vi "Simulation iRobot Sensors.vi"(8 "error in":errorcluster, 11 "simulator":T11={"configuration"={"maxTime"=5.0, "enableVisualization"=TRUE, "statechart"=path "iRobot Navigation State Machine.vi", "environment"=path "simulation configuration.ini", "record"=path "Simulation Record.xml", "autograde?"=TRUE, "interactive?"=FALSE, "feedback mode"=enum."debug navigation"}, "Bump Sensors"=[], "Distance Sensors"=[], "Accelerometer"=refnum, "Wall Sensor"=refnum, "Statechart\ndisplay"=refnum, "Body"=refnum, "Left Motor"=refnum, "Right Motor"=refnum, "first step?"=FALSE}) -> (0 "error out":errorcluster, 2 "sensors":T1={"net distance (mm)"=0, "net angle (deg)"=0, "accelerometer"={"x axis (g)"=0.0, "y axis (g)"=0.0, "z axis (g)"=0.0}, "iRobot Sensors"={"Bumps + Wheel Drops"={"Wheeldrop Caster"=FALSE, "Wheeldrop Left"=FALSE, "Wheeldrop Right"=FALSE, "Bump Left"=FALSE, "Bump Right"=FALSE}, "Wall"=FALSE, "Cliff Left"=FALSE, "Cliff Front Left"=FALSE, "Cliff Front Right"=FALSE, "Cliff Right"=FALSE, "Wall Signal"=0, "Cliff Left Signal"=0, "Cliff Front Left Signal"=0, "Cliff Front Right Signal"=0, "Cliff Right Signal"=0, "Buttons"={"Advance"=FALSE, "Play"=FALSE}, "Virtual Wall"=FALSE, "# Stream Packets"=0, "Requested Velocity (mm/s)"=0, "Requested Radius (mm)"=0, "Requested Right Wheel Velocity (mm/s)"=0, "Requested Left Wheel Velocity (mm/s)"=0, "Distance (mm)"=0, "Angle (deg)"=0, "Song Playing"=FALSE, "Song Number"=0, "Charging State"=enum."Not Charging", "Voltage (mV)"=0, "Current (mA)"=0, "Battery Temperature (deg C)"=0, "Battery Charge (mAh)"=0, "Battery Capacity (mAh)"=0, "Charging Sources"={"Internal Charger"=FALSE, "Home Base"=FALSE}, "OI Mode"=enum."Off", "Digital Inputs"={"Digital Input 0"=FALSE, "Digital Input 1"=FALSE, "Digital Input 2"=FALSE, "Digital Input 3"=FALSE, "Device Detect"=FALSE}, "Drivers & Wheel Overcurrent"={"Low-Side Driver 0"=FALSE, "Low-Side Driver 1"=FALSE, "Low-Side Driver 2"=FALSE, "Left Wheel"=FALSE, "Right Wheel"=FALSE}, "Analog Signal"=0, "Infrared"=255}, "Is Simulator?"=FALSE} {"iRobot Sensors"."Infrared" format="%02x"; "accelerometer"."z axis (g)" format="%.3f"; "accelerometer"."y axis (g)" format="%.3f"; "accelerometer"."x axis (g)" format="%.3f"}, 3 "simulator":T11={"configuration"={"maxTime"=5.0, "enableVisualization"=TRUE, "statechart"=path "iRobot Navigation State Machine.vi", "environment"=path "simulation configuration.ini", "record"=path "Simulation Record.xml", "autograde?"=TRUE, "interactive?"=FALSE, "feedback mode"=enum."debug navigation"}, "Bump Sensors"=[], "Distance Sensors"=[], "Accelerometer"=refnum, "Wall Sensor"=refnum, "Statechart\ndisplay"=refnum, "Body"=refnum, "Left Motor"=refnum, "Right Motor"=refnum, "first step?"=FALSE})   [LabVIEW 2013]
doc: "Simulates iRobot sensors. Automatically accumulates distance and angle."
uses:
  Simulator.ctl
  <instrlib>/DC Motor Controller/HAIOL/DC Motor Controller.lvclass
  CyberSim interface/Simulation Configuration.ctl
  autograder/feedbackMode.ctl
  shared/Sensors.ctl
  iRobot/Sensor/Accelerometer.ctl
  iRobot/Sensor/Sensor Group 6.ctl
  iRobot/Sensor/Bumps + Wheel Drops.ctl
  iRobot/Sensor/Buttons.ctl
  iRobot/Sensor/Charging State.ctl
  iRobot/Sensor/Charging Sources Available.ctl
  iRobot/Sensor/OI Mode.ctl
  iRobot/Sensor/Cargo Bay Digital Inputs.ctl
  iRobot/Sensor/Low-Side Driver + Wheel Overcurrent.ctl
  <vilib>/Analysis/coordinate.llb/Angle Units.ctl
  <vilib>/Analysis/coordinate.llb/Wrap Angle (scalar).vi
  <vilib>/Analysis/coordinate.llb/2D Cartesian Coordinate Rotation (Scalar).vi
  <vilib>/Analysis/BLAS.llb/dnrm2 - Vector 2-Norm (DBL).vi
  <resource>/objmgr/LVODE.rc
  <vilib>/Analysis/NI_AALBLAS.lvlib
  <vilib>/robotics/Kinematics/NI_Kinematics.lvlib
  <vilib>/Analysis/NI_AAL_Angle.lvlib
  <vilib>/Analysis/NI_AALPro.lvlib
panel:
  # "Electrical: charging, battery, OI mode"
  # "Sensors: bump, cliff, button, wheel drop, wall, virtual wall"
  # "Motion: distance, angle, requested velocity"
  # "Cargo Bay: I/O, overcurrent, infrared"
  # "Song"
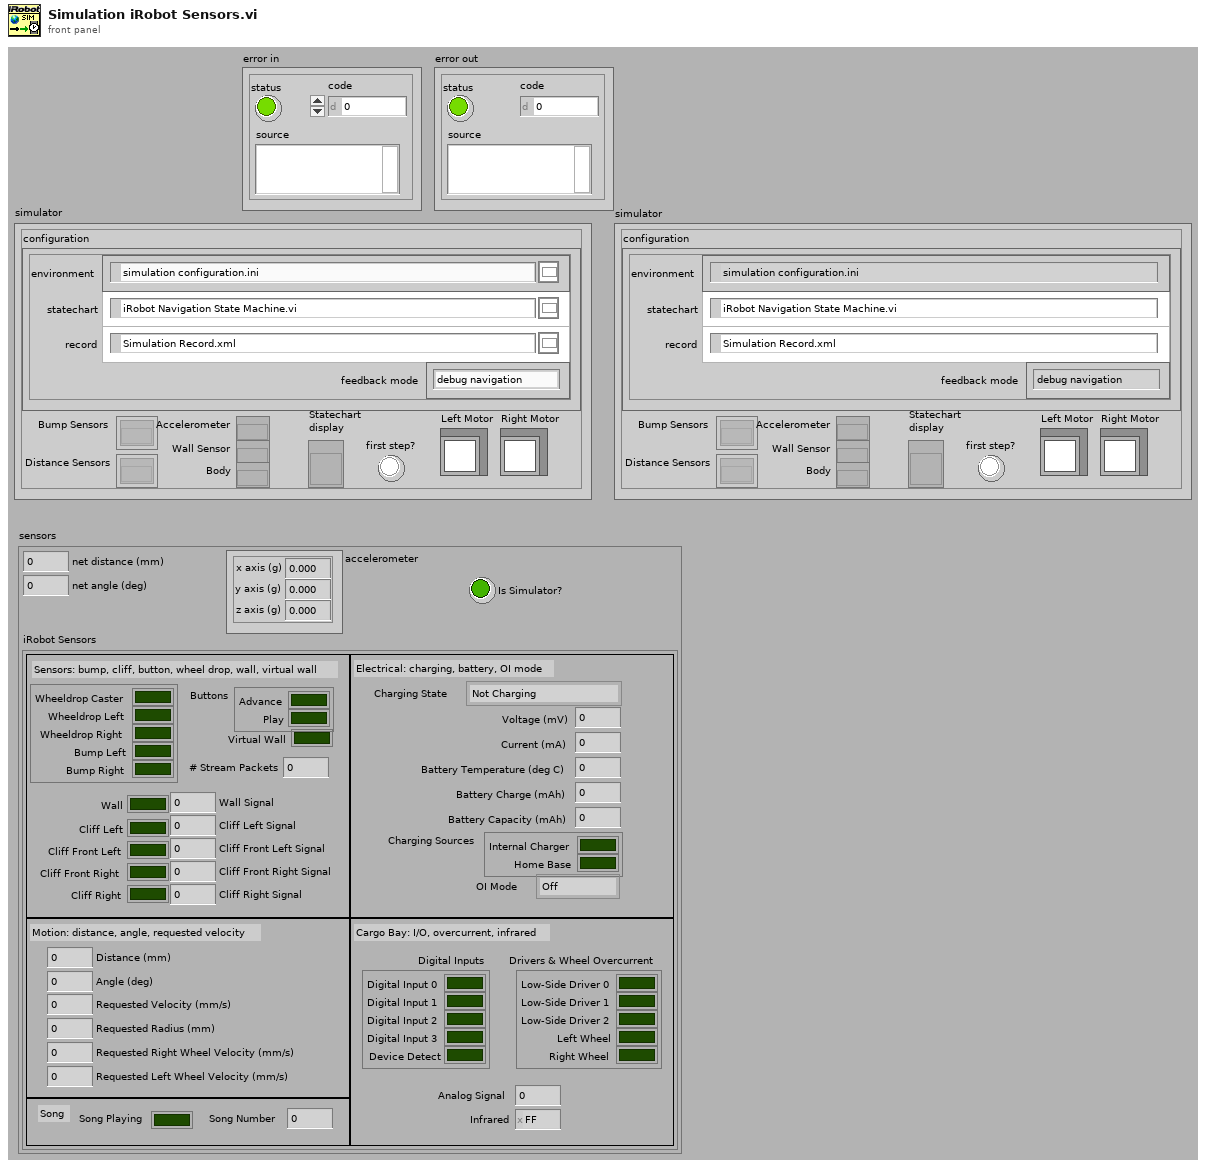
[diagram p1: front panel]
types:
  T1 = typedef "Sensors.ctl" = cluster{"net distance (mm)":i32, "net angle (deg)":i32, "accelerometer":T2, "iRobot Sensors":T3, "Is Simulator?":bool}
  T2 = typedef "Accelerometer.ctl" = cluster{"x axis (g)":dbl, "y axis (g)":dbl, "z axis (g)":dbl}
  T3 = typedef "Sensor Group 6.ctl" = cluster{"Bumps + Wheel Drops":T4, "Wall":bool, "Cliff Left":bool, "Cliff Front Left":bool, "Cliff Front Right":bool, "Cliff Right":bool, "Wall Signal":u16, "Cliff Left Signal":u16, "Cliff Front Left Signal":u16, "Cliff Front Right Signal":u16, "Cliff Right Signal":u16, "Buttons":T5, "Virtual Wall":bool, "# Stream Packets":u8, "Requested Velocity (mm/s)":i16, "Requested Radius (mm)":i16, "Requested Right Wheel Velocity (mm/s)":i16, "Requested Left Wheel Velocity (mm/s)":i16, "Distance (mm)":i32, "Angle (deg)":i32, "Song Playing":bool, "Song Number":u8, "Charging State":T6, "Voltage (mV)":u16, "Current (mA)":i16, "Battery Temperature (deg C)":i8, "Battery Charge (mAh)":u16, "Battery Capacity (mAh)":u16, "Charging Sources":T7, "OI Mode":T8, "Digital Inputs":T9, "Drivers & Wheel Overcurrent":T10, "Analog Signal":u16, "Infrared":u8}
  T4 = typedef "Bumps + Wheel Drops.ctl" = cluster{"Wheeldrop Caster":bool, "Wheeldrop Left":bool, "Wheeldrop Right":bool, "Bump Left":bool, "Bump Right":bool}
  T5 = typedef "Buttons.ctl" = cluster{"Advance":bool, "Play":bool}
  T6 = typedef "Charging State.ctl" = enum16{"Not Charging", "Reconditioning Charging", "Full Charging", "Trickle Charging", "Waiting", "Charging Fault Condition"}
  T7 = typedef "Charging Sources Available.ctl" = cluster{"Internal Charger":bool, "Home Base":bool}
  T8 = typedef "OI Mode.ctl" = enum16{"Off", "Passive", "Safe", "Full"}
  T9 = typedef "Cargo Bay Digital Inputs.ctl" = cluster{"Digital Input 0":bool, "Digital Input 1":bool, "Digital Input 2":bool, "Digital Input 3":bool, "Device Detect":bool}
  T10 = typedef "Low-Side Driver + Wheel Overcurrent.ctl" = cluster{"Low-Side Driver 0":bool, "Low-Side Driver 1":bool, "Low-Side Driver 2":bool, "Left Wheel":bool, "Right Wheel":bool}
  T11 = typedef "Simulator.ctl" = cluster{"configuration":T12, "Bump Sensors":refnum<k20>[], "Distance Sensors":refnum<k20>[], "Accelerometer":refnum<k20>, "Wall Sensor":refnum<k20>, "Statechart\ndisplay":refnum<vi>, "Body":refnum<k20>, "Left Motor":refnum<class "DC Motor Controller.lvclass">, "Right Motor":refnum<class "DC Motor Controller.lvclass">, "first step?":bool}
  T12 = typedef "Simulation Configuration.ctl" = cluster{"maxTime":sgl, "enableVisualization":bool, "statechart":path, "environment":path, "record":path, "autograde?":bool, "interactive?":bool, "feedback mode":T13}
  T13 = typedef "feedbackMode.ctl" = enum32{"debug navigation", "debug hill climb", "autograde navigation", "autograde hill climb"}
  T14 = typedef "NI_AAL_Angle.lvlib/Angle Units.ctl" = i32
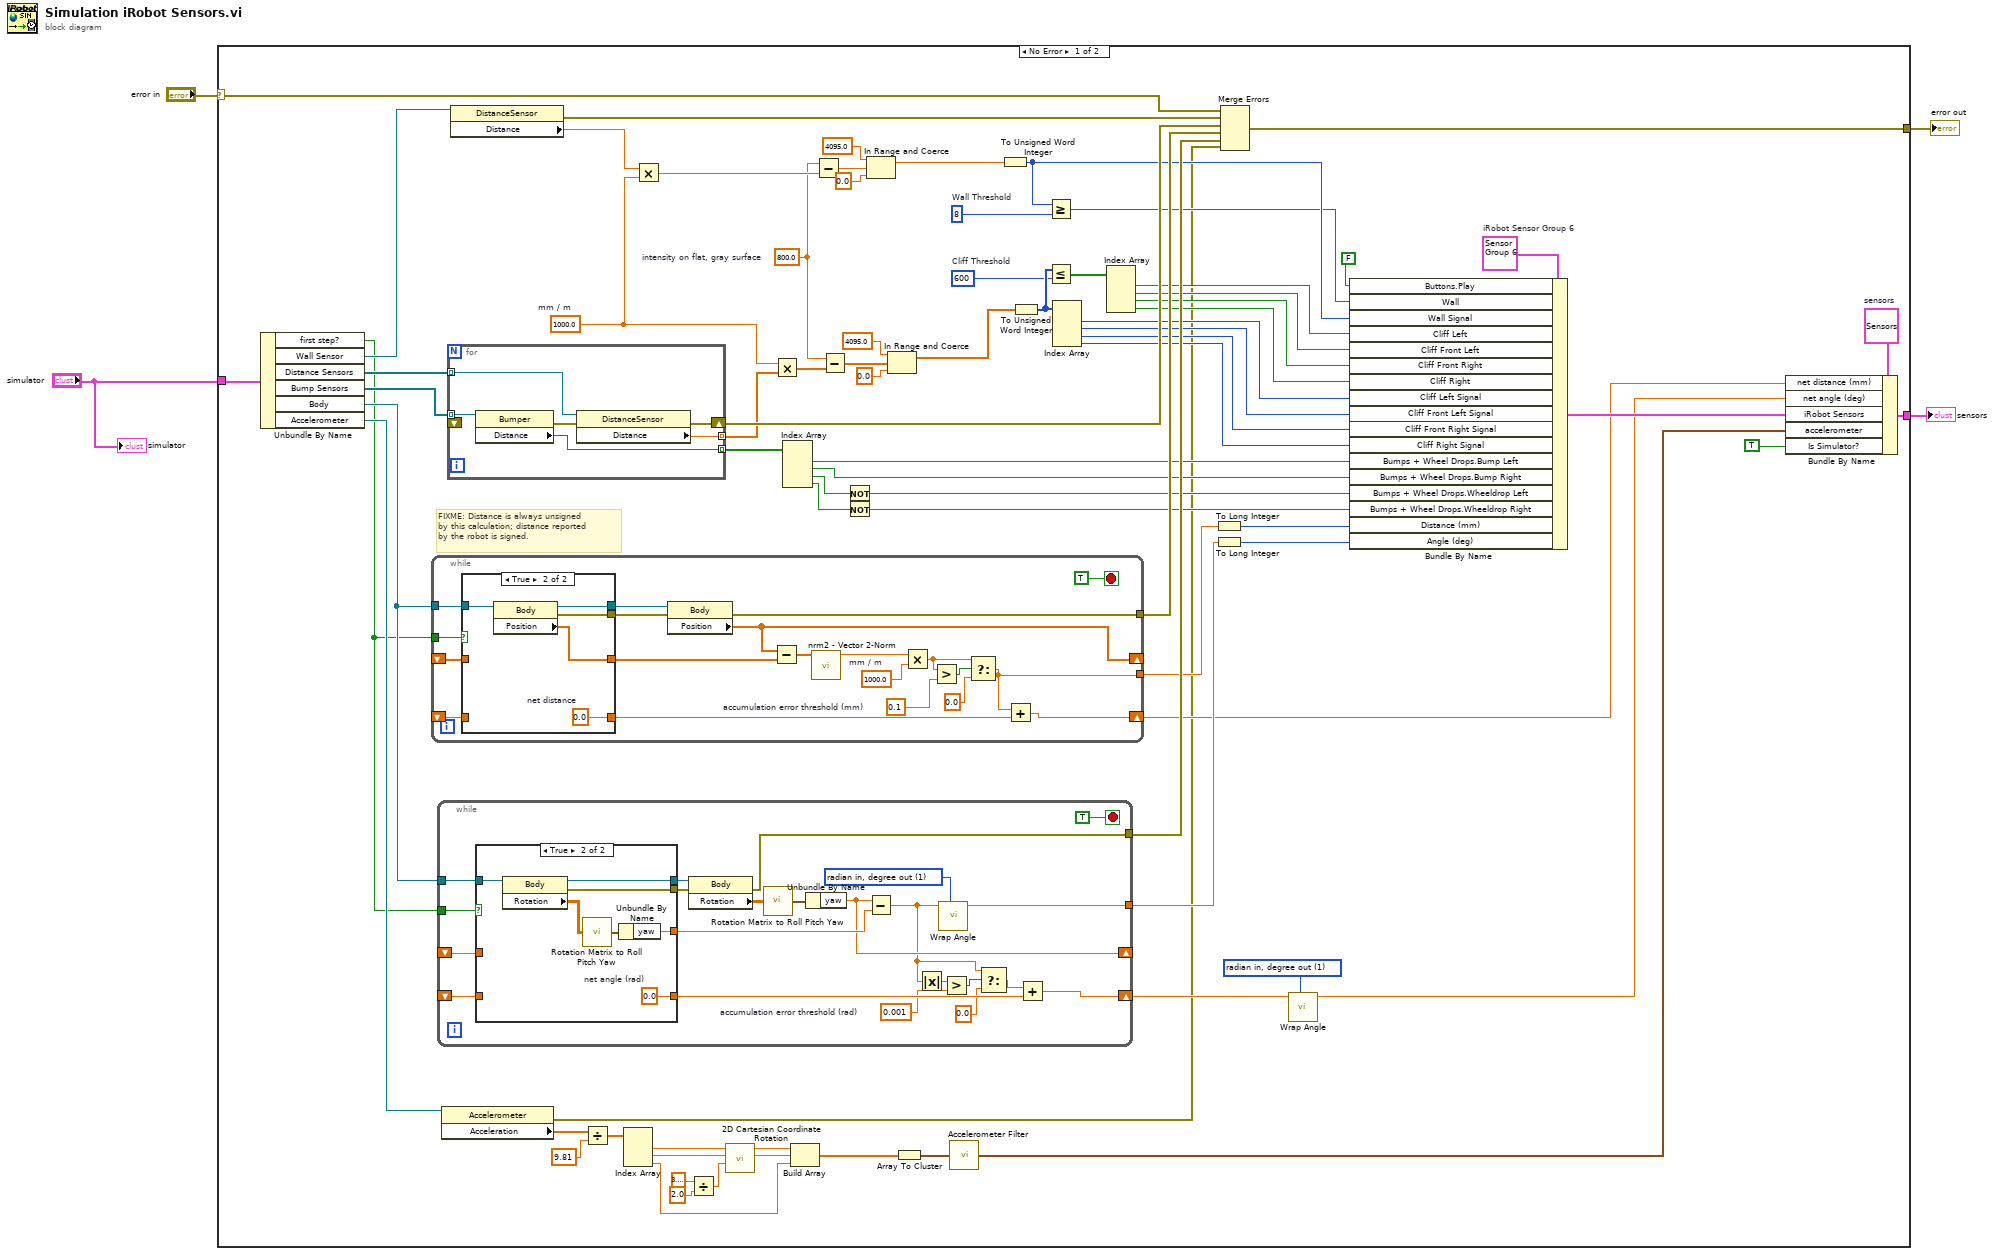
[diagram p0: block diagram]
diagram:
  n1 = case shown="No Error" "error in" {
    selector: "error in" -> [w8 w148]
    tunnel: [w14 _] -> w4
    tunnel: "simulator" -> [w12 _]
    tunnel: [w9 w148] -> w2
    frame No Error {
      w15 = T1 {"net distance (mm)"=0, "net angle (deg)"=0, "accelerometer"={"x axis (g)"=0.0, "y axis (g)"=0.0, "z axis (g)"=0.0}, "iRobot Sensors"={"Bumps + Wheel Drops"={"Wheeldrop Caster"=FALSE, "Wheeldrop Left"=FALSE, "Wheeldrop Right"=FALSE, "Bump Left"=FALSE, "Bump Right"=FALSE}, "Wall"=FALSE, "Cliff Left"=FALSE, "Cliff Front Left"=FALSE, "Cliff Front Right"=FALSE, "Cliff Right"=FALSE, "Wall Signal"=0, "Cliff Left Signal"=0, "Cliff Front Left Signal"=0, "Cliff Front Right Signal"=0, "Cliff Right Signal"=0, "Buttons"={"Advance"=FALSE, "Play"=FALSE}, "Virtual Wall"=FALSE, "# Stream Packets"=0, "Requested Velocity (mm/s)"=0, "Requested Radius (mm)"=0, "Requested Right Wheel Velocity (mm/s)"=0, "Requested Left Wheel Velocity (mm/s)"=0, "Distance (mm)"=0, "Angle (deg)"=0, "Song Playing"=FALSE, "Song Number"=0, "Charging State"=enum."Not Charging", "Voltage (mV)"=0, "Current (mA)"=0, "Battery Temperature (deg C)"=0, "Battery Charge (mAh)"=0, "Battery Capacity (mAh)"=0, "Charging Sources"={"Internal Charger"=FALSE, "Home Base"=FALSE}, "OI Mode"=enum."Off", "Digital Inputs"={"Digital Input 0"=FALSE, "Digital Input 1"=FALSE, "Digital Input 2"=FALSE, "Digital Input 3"=FALSE, "Device Detect"=FALSE}, "Drivers & Wheel Overcurrent"={"Low-Side Driver 0"=FALSE, "Low-Side Driver 1"=FALSE, "Low-Side Driver 2"=FALSE, "Left Wheel"=FALSE, "Right Wheel"=FALSE}, "Analog Signal"=0, "Infrared"=0}, "Is Simulator?"=FALSE}  # sensors
      w40 = u16 8  # Wall Threshold
      w41 = 800.0  # intensity on flat, gray surface
      w45 = T14 1 items=["radian in, radian out", "radian in, degree out", "degree in, degree out", "degree in, radian out"] ("angle units")
      w49 = 600  # Cliff Threshold
      w69 = T3 {"Bumps + Wheel Drops"={"Wheeldrop Caster"=FALSE, "Wheeldrop Left"=FALSE, "Wheeldrop Right"=FALSE, "Bump Left"=FALSE, "Bump Right"=FALSE}, "Wall"=FALSE, "Cliff Left"=FALSE, "Cliff Front Left"=FALSE, "Cliff Front Right"=FALSE, "Cliff Right"=FALSE, "Wall Signal"=0, "Cliff Left Signal"=0, "Cliff Front Left Signal"=0, "Cliff Front Right Signal"=0, "Cliff Right Signal"=0, "Buttons"={"Advance"=FALSE, "Play"=FALSE}, "Virtual Wall"=FALSE, "# Stream Packets"=0, "Requested Velocity (mm/s)"=0, "Requested Radius (mm)"=0, "Requested Right Wheel Velocity (mm/s)"=0, "Requested Left Wheel Velocity (mm/s)"=0, "Distance (mm)"=0, "Angle (deg)"=0, "Song Playing"=FALSE, "Song Number"=0, "Charging State"=enum."Not Charging", "Voltage (mV)"=0, "Current (mA)"=0, "Battery Temperature (deg C)"=0, "Battery Charge (mAh)"=0, "Battery Capacity (mAh)"=0, "Charging Sources"={"Internal Charger"=FALSE, "Home Base"=FALSE}, "OI Mode"=enum."Off", "Digital Inputs"={"Digital Input 0"=FALSE, "Digital Input 1"=FALSE, "Digital Input 2"=FALSE, "Digital Input 3"=FALSE, "Device Detect"=FALSE}, "Drivers & Wheel Overcurrent"={"Low-Side Driver 0"=FALSE, "Low-Side Driver 1"=FALSE, "Low-Side Driver 2"=FALSE, "Left Wheel"=FALSE, "Right Wheel"=FALSE}, "Analog Signal"=0, "Infrared"=0}  # iRobot Sensor Group 6
      w74 = 1000.0  # mm / m
      # "FIXME: Distance is always unsigned\nby this calculation; distance reported\nby the robot is signed."
      n2 = Unbundle By Name(w12) -> ("first step?"=w6:bool, "Wall Sensor"=w79:refnum<k20>, "Distance Sensors"=w80:refnum<k20>[], "Bump Sensors"=w81:refnum<k20>[], "Body"=w44:refnum<k20>, "Accelerometer"=w31:refnum<k20>)
      n3 = while {
        tunnel: w44 -> [w133]
        shift-right: [w122] -> _
        shift-left: _ -> [w132]
        tunnel: [w128] -> w71
        shift-right: [w123] -> w17
        shift-left: _ -> [w121]
        tunnel: [w115] -> w58
        tunnel: w6 -> [w114]
        stop <- TRUE stop-if-true
        w117 = 0.1  # accumulation error threshold (mm)
        w125 = 1000.0  # mm / m
        n4 = case shown="True" w114 {
          tunnel: w133 -> [w135 w141]
          tunnel: [w136 w138] -> w127
          tunnel: w132 -> [w136 _]
          tunnel: [_ w140] -> w129
          tunnel: [w135 w139] -> w130
          tunnel: w121 -> [w134 _]
          tunnel: [w134 w137] -> w120
          frame False {
          }
          frame True {
            w137 = 0.0  # net distance
            n5 = property class="Body"(reference=w141) -> (reference out=w139:refnum<k20>, error out=w140:errorcluster, "Position"=w138:sgl[])  [unwired: 1 in]
          }
        }
        n6 = property class="Body"(reference=w130, error in=w129) -> (error out=w128:errorcluster, "Position"=w122:sgl[])  [unwired: 1 out]
        n7 = Subtract(x=w122, y=w127) -> (x-y=w124:sgl[])
        n8 = call-poly <vilib>:"nrm2 - Vector 2-Norm.vi"("x"=w124) -> ("dnrm2"=w126:dbl)  [unwired: 9 in, 1 out]
        n9 = Multiply(x=w126, y=w125) -> (x*y=w119:dbl)
        n10 = Greater?(x=w119, y=w117) -> (0:w118:bool)
        n11 = Select(t=w119, s=w118, f=0.0) -> (s? t:f=w115:dbl)
        n12 = Add(x=w115, y=w120) -> (x+y=w123:dbl)
      }
      n13 = while {
        tunnel: w44 -> [w102]
        tunnel: [w96] -> w70
        tunnel: [w83] -> w56
        shift-right: [w86] -> _
        shift-left: _ -> [w95]
        shift-right: [w93] -> w46
        shift-left: _ -> [w94]
        tunnel: w6 -> [w82]
        stop <- TRUE stop-if-true
        w84 = T14 1 items=["radian in, radian out", "radian in, degree out", "degree in, degree out", "degree in, radian out"] ("angle units")
        w88 = 0.001  # accumulation error threshold (rad)
        n14 = case shown="True" w82 {
          tunnel: w102 -> [w106 w113]
          tunnel: [w106 w112] -> w101
          tunnel: [_ w111] -> w100
          tunnel: [w105 w108] -> w97
          tunnel: w95 -> [w105 _]
          tunnel: [w104 w107] -> w90
          tunnel: w94 -> [w104 _]
          frame False {
          }
          frame True {
            w107 = 0.0  # net angle (rad)
            n15 = property class="Body"(reference=w113) -> (reference out=w112:refnum<k20>, error out=w111:errorcluster, "Rotation"=w110:sgl[][])  [unwired: 1 in]
            n16 = call <vilib>:"Rotation Matrix to Roll Pitch Yaw.vi"("rotation matrix"=w110) -> ("angles"=w109:cluster{"roll":dbl, "pitch":dbl, "yaw":dbl})
            n17 = Unbundle By Name(w109) -> ("yaw"=w108:dbl)
          }
        }
        n18 = property class="Body"(reference=w101, error in=w100) -> (error out=w96:errorcluster, "Rotation"=w99:sgl[][])  [unwired: 1 out]
        n19 = call <vilib>:"Rotation Matrix to Roll Pitch Yaw.vi"("rotation matrix"=w99) -> ("angles"=w98:cluster{"roll":dbl, "pitch":dbl, "yaw":dbl})
        n20 = Unbundle By Name(w98) -> ("yaw"=w86:dbl)
        n21 = Subtract(x=w86, y=w97) -> (x-y=w85:dbl)
        n22 = Absolute Value(x=w85) -> (abs(x)=w87:dbl)
        n23 = call-poly <vilib>:"Wrap Angle.vi"("angle units"=w84, "angle in"=w85) -> ("angle out"=w83:dbl)  [unwired: 8 in, 1 out]
        n24 = Greater?(x=w87, y=w88) -> (0:w92:bool)
        n25 = Select(t=w85, s=w92, f=0.0) -> (s? t:f=w91:dbl)
        n26 = Add(x=w91, y=w90) -> (x+y=w93:dbl)
      }
      n27 = property class="Accelerometer"(reference=w31) -> (error out=w7:errorcluster, "Acceleration"=w30:sgl[])  [unwired: 1 in, 1 out]
      n28 = for {
        tunnel: [w147] -> w64 mode=indexing
        tunnel: w81 -> [w146] mode=indexing
        tunnel: [w145] -> w75 mode=indexing
        shift-right: [w143] -> w72
        shift-left: _ -> [_]
        tunnel: w80 -> [w142] mode=indexing
        n29 = property class="Bumper"(reference=w146) -> (error out=w144:errorcluster, "Distance"=w145:bool)  [unwired: 1 in, 1 out]
        n30 = property class="DistanceSensor"(reference=w142, error in=w144) -> (error out=w143:errorcluster, "Distance"=w147:sgl)  [unwired: 1 out]
      }
      n31 = property class="DistanceSensor"(reference=w79) -> (error out=w73:errorcluster, "Distance"=w78:sgl)  [unwired: 1 in, 1 out]
      n32 = Divide(x=w30, y=9.81) -> (x/y=w28:dbl[])
      n33 = Index Array(array=w28) -> (element #1=w27:dbl, element #2=w26:dbl, element #3=w20:dbl)  [unwired: 3 in]
      n34 = Multiply(x=w78, y=w74) -> (x*y=w42:dbl)
      n35 = Divide(x=3.141592653589793, y=2.0) -> (x/y=w23:dbl)
      n36 = call-poly <vilib>:"2D Cartesian Coordinate Rotation.vi"("theta"=w23, "y"=w26, "x"=w27) -> ("y out"=w21:dbl, "x out"=w22:dbl)  [unwired: 6 in, 1 out]
      n37 = Multiply(x=w74, y=w64) -> (x*y=w43:dbl[])
      n38 = Index Array(array=w75) -> (element #1=w68:bool, element #2=w67:bool, element #3=w77:bool, element #4=w76:bool)  [unwired: 4 in]
      n39 = Build Array(w22, w21, w20) -> (w19:dbl[])
      n40 = Subtract(x=w41, y=w42) -> (x-y=w39:dbl)
      n41 = Subtract(x=w41, y=w43) -> (x-y=w33:dbl[])
      n42 = Not(x=w77) -> (.not. x?=w66:bool)
      n43 = Not(x=w76) -> (.not. x?=w65:bool)
      n44 = In Range and Coerce(upper limit=4095.0, x=w39, lower limit=0.0) -> (coerced(x)=w36:dbl)  [unwired: 1 out]
      n45 = In Range and Coerce(upper limit=4095.0, x=w33, lower limit=0.0) -> (coerced(x)=w32:dbl[])  [unwired: 1 out]
      n46 = Array To Cluster(array=w19) -> (cluster=w11:cluster{"[0]":dbl, "[1]":dbl, "[2]":dbl})
      n47 = call "Accelerometer Filter.vi"("accelerometer (g)"=w11) -> ("filtered accelerometer (g)"=w10:T2)  [unwired: 3 in]
      n48 = To Unsigned Word Integer(number=w36) -> (unsigned 16bit integer=w48:u16)
      n49 = To Unsigned Word Integer(number=w32) -> (unsigned 16bit integer=w55:u16[])
      n50 = Greater Or Equal?(x=w48, y=w40) -> (x >= y?=w47:bool)
      n51 = Less Or Equal?(x=w55, y=w49) -> (x <= y?=w54:bool[])
      n52 = Index Array(array=w55) -> (element #1=w63:u16, element #2=w62:u16, element #3=w61:u16, element #4=w60:u16)  [unwired: 4 in]
      n53 = Index Array(array=w54) -> (element #1=w50:bool, element #2=w51:bool, element #3=w52:bool, element #4=w53:bool)  [unwired: 4 in]
      n54 = To Long Integer(number=w58) -> (32bit integer=w59:i32)
      n55 = To Long Integer(number=w56) -> (32bit integer=w57:i32)
      n56 = Merge Errors(w8, w73, w72, w71, w70, w7) -> (w9:errorcluster)
      n57 = call-poly <vilib>:"Wrap Angle.vi"("angle units"=w45, "angle in"=w46) -> ("angle out"=w16:dbl)  [unwired: 8 in, 1 out]
      n58 = Bundle By Name(cluster=w69, "Buttons.Play"=FALSE, "Wall"=w47, "Wall Signal"=w48, "Cliff Left"=w50, "Cliff Front Left"=w51, "Cliff Front Right"=w52, "Cliff Right"=w53, "Cliff Left Signal"=w63, "Cliff Front Left Signal"=w62, "Cliff Front Right Signal"=w61, "Cliff Right Signal"=w60, "Bumps + Wheel Drops.Bump Left"=w68, "Bumps + Wheel Drops.Bump Right"=w67, "Bumps + Wheel Drops.Wheeldrop Left"=w66, "Bumps + Wheel Drops.Wheeldrop Right"=w65, "Distance (mm)"=w59, "Angle (deg)"=w57) -> (w18:T3)
      n59 = Bundle By Name(cluster=w15, "net distance (mm)"=w17, "net angle (deg)"=w16, "iRobot Sensors"=w18, "accelerometer"=w10, "Is Simulator?"=TRUE) -> (w14:T1)
    }
    frame Error {
    }
  }
  "error out" <- w2
  "sensors" <- w4
  "simulator" <- "simulator"
